vi "test9cameras.vi"() -> ()   [LabVIEW 2013]
uses:
  <vilib>/vision/Image Controls.llb/IMAQ Image.ctl
  shared programs/GUI_Template/GUI_master/tcp new data cluster.ctl
  shared programs/GUI_Template/GUI_master/tcp_new_data_event.ctl
panel:
  in  "names1":bool
  in  "MirrorsNames 2":string[](array[string])=["TS-253a_in"]
  out "image::6":T1(plugin-control) caption="Mode1"
  out "image::5":T1(plugin-control) caption="Mode1"
  out "image::4":T1(plugin-control) caption="Mode1"
  out "image::3":T1(plugin-control) caption="Mode1"
  out "image::2":T1(plugin-control) caption="Mode1"
  out "error IO 2":errorcluster
  in  "insert tag":bool=TRUE
  out "tcp data event":T2
  out "GUIdevice 1":string="M1Cam"
  out "GUIdevice 2":string="M1Cam"
  out "GUIdevice 3":string="M1Cam"
  out "GUIdevice 4":string="M1Cam"
  out "GUIdevice 5":string="M1Cam"
  out "GUIdevice 6":string="M1Cam"
  out "image::1":T1(plugin-control) caption="Mode1"
  in  "MirrorsNames":string[](array[string])=["TS-253a_in", "TS-Mode1", "StagingAlignBeam1", "StagingM1Far", "StagingM1Near", "StagingM3Far", "StagingOAP1Far", "StagingOAP1Near", "StagingOAP2Near"]
  in  "stop":bool
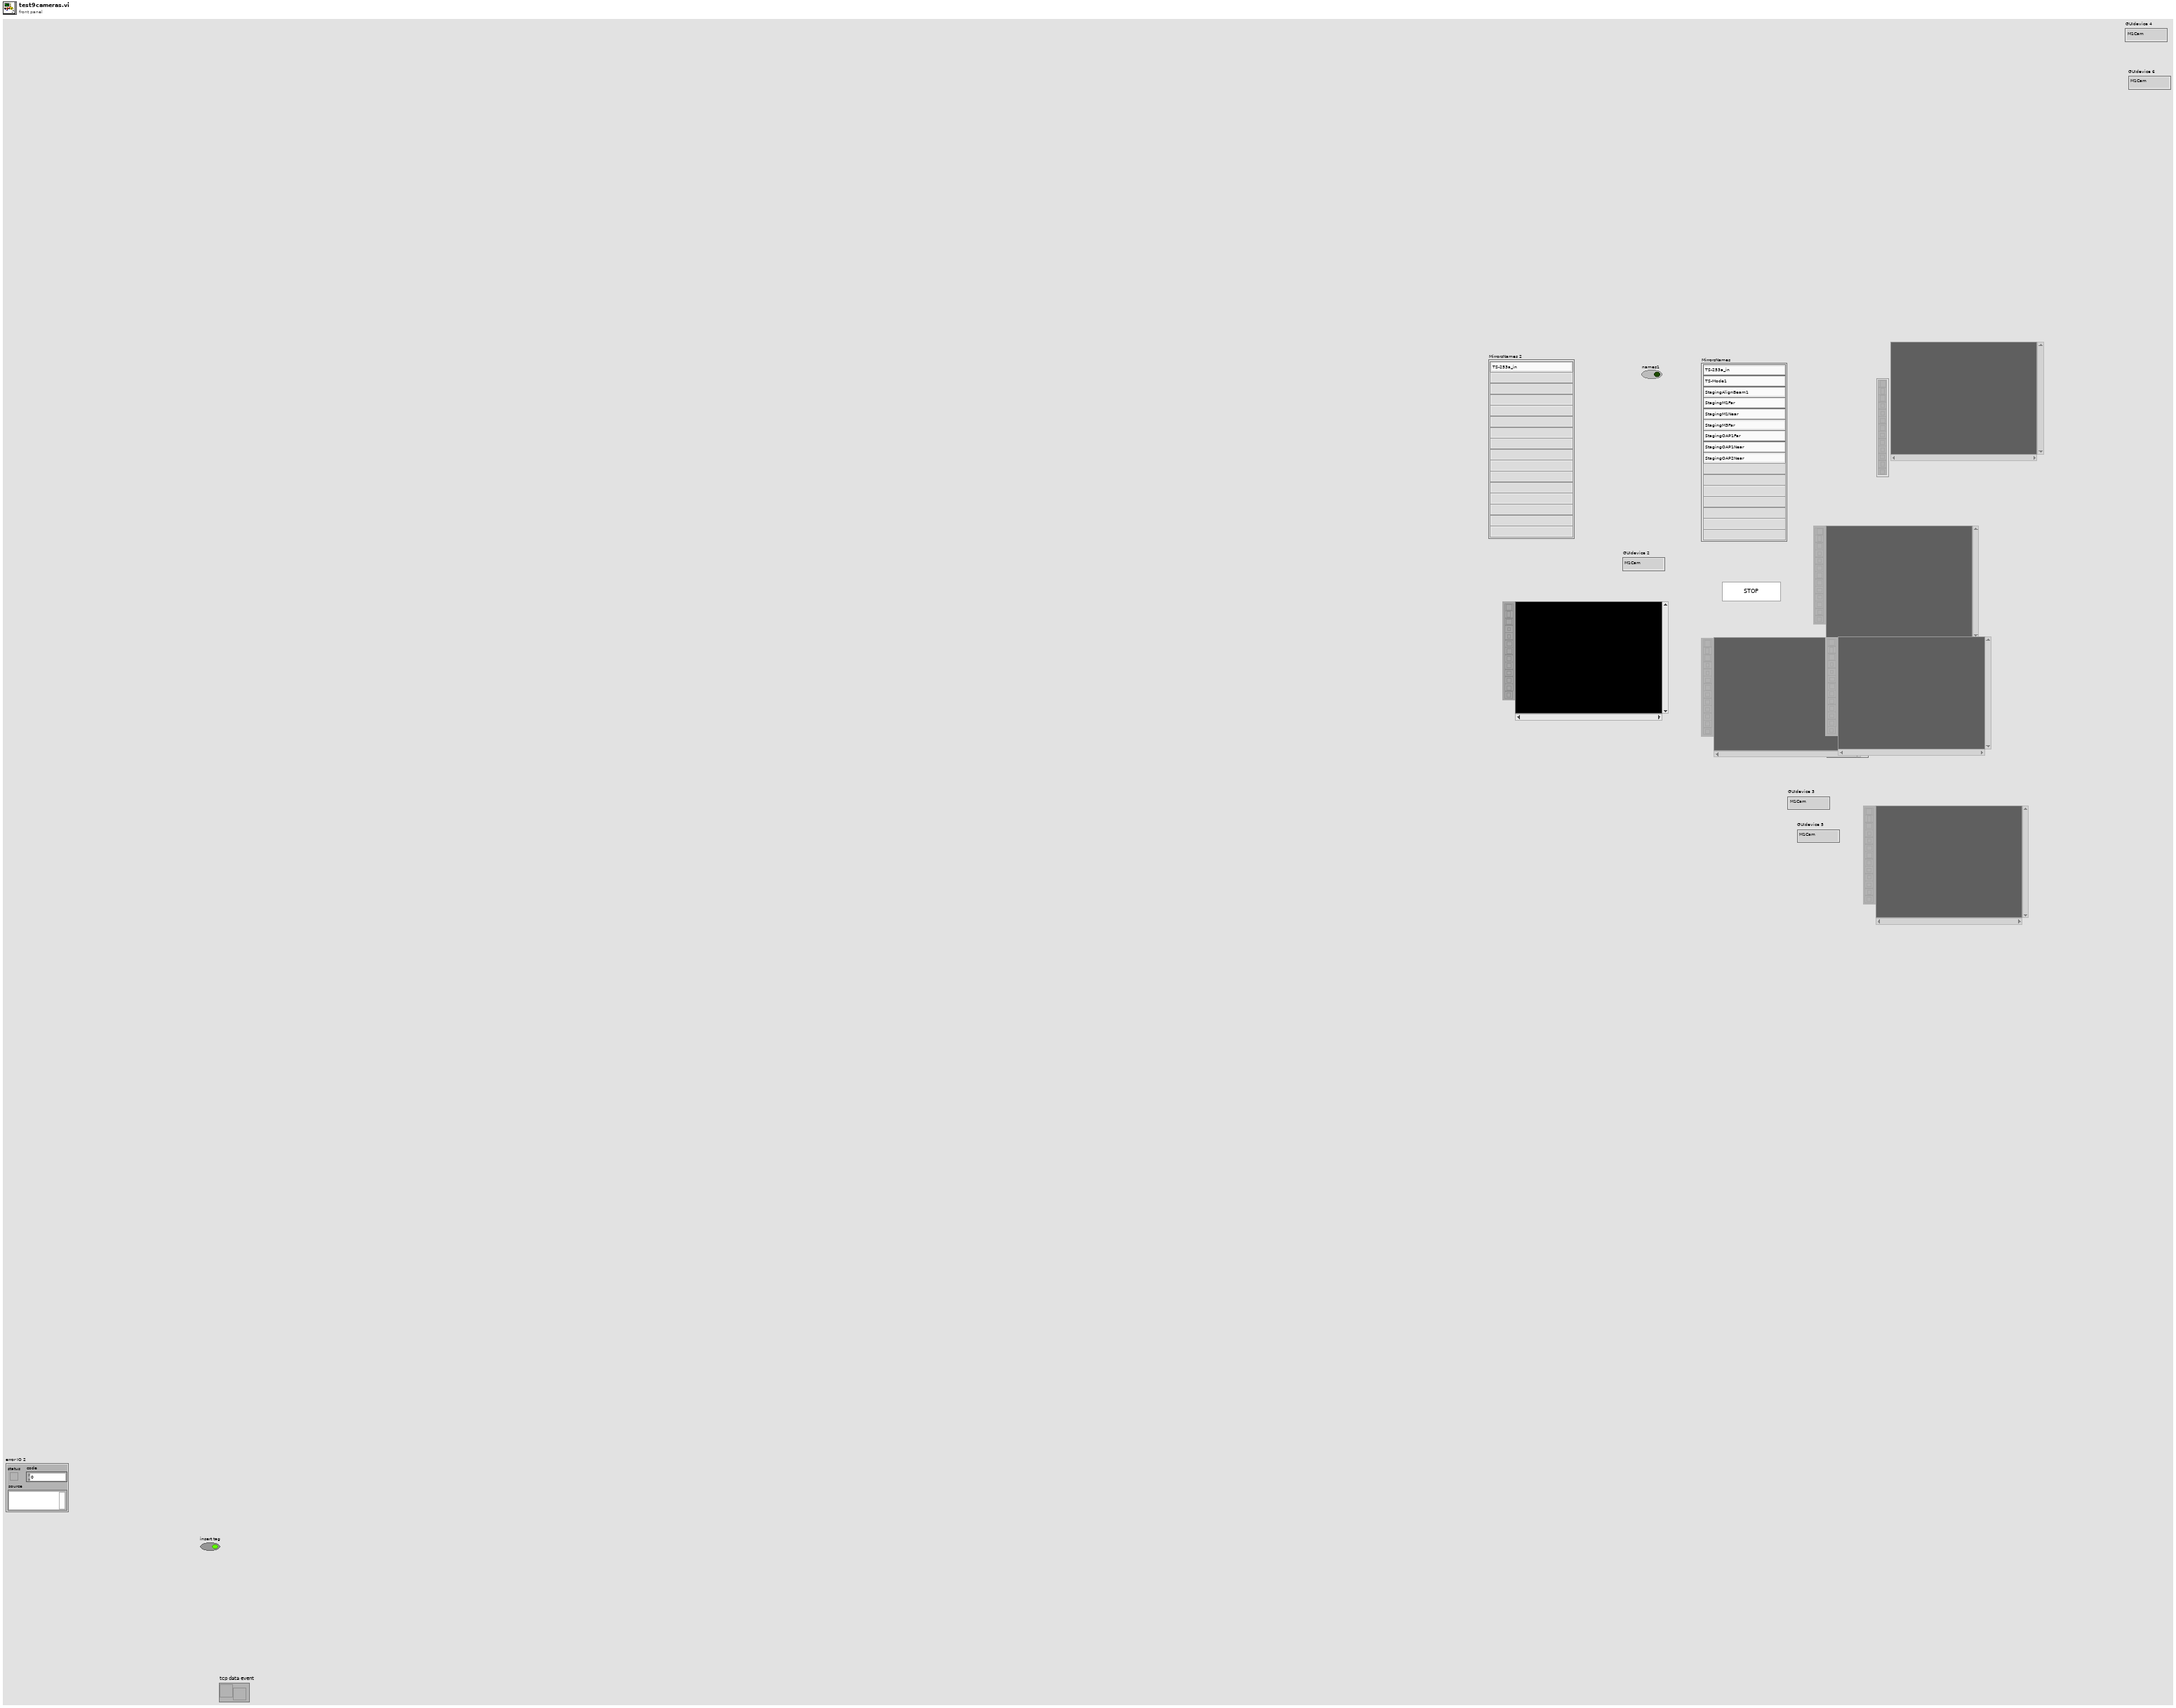
[diagram p1: front panel]
types:
  T1 = typedef "IMAQ Image.ctl" = refnum<image>
  T2 = typedef "tcp_new_data_event.ctl" = refnum<user-event>
  T3 = enum32{"invalid app kind", "Development System", "Run Time System", "Student Edition", "Embedded LabVIEW", "Evaluation", "Custom"}
  T4 = enum32{"Invalid", "Standard", "Closed", "Hidden", "Minimized", "Maximized"}
  T5 = cluster{"Core":cluster{"Current VI Reference":refnum<vi>, "Close Panel on Exit?":bool}, "Your Boolean data":bool, "Your string data":string}
  T6 = cluster{"Current VI Reference":refnum<vi>, "Close Panel on Exit?":bool}
  T7 = typedef "tcp new data cluster.ctl" = cluster{"EventEnum":enum16{"new data", "connection status update"}, "Device name":string}
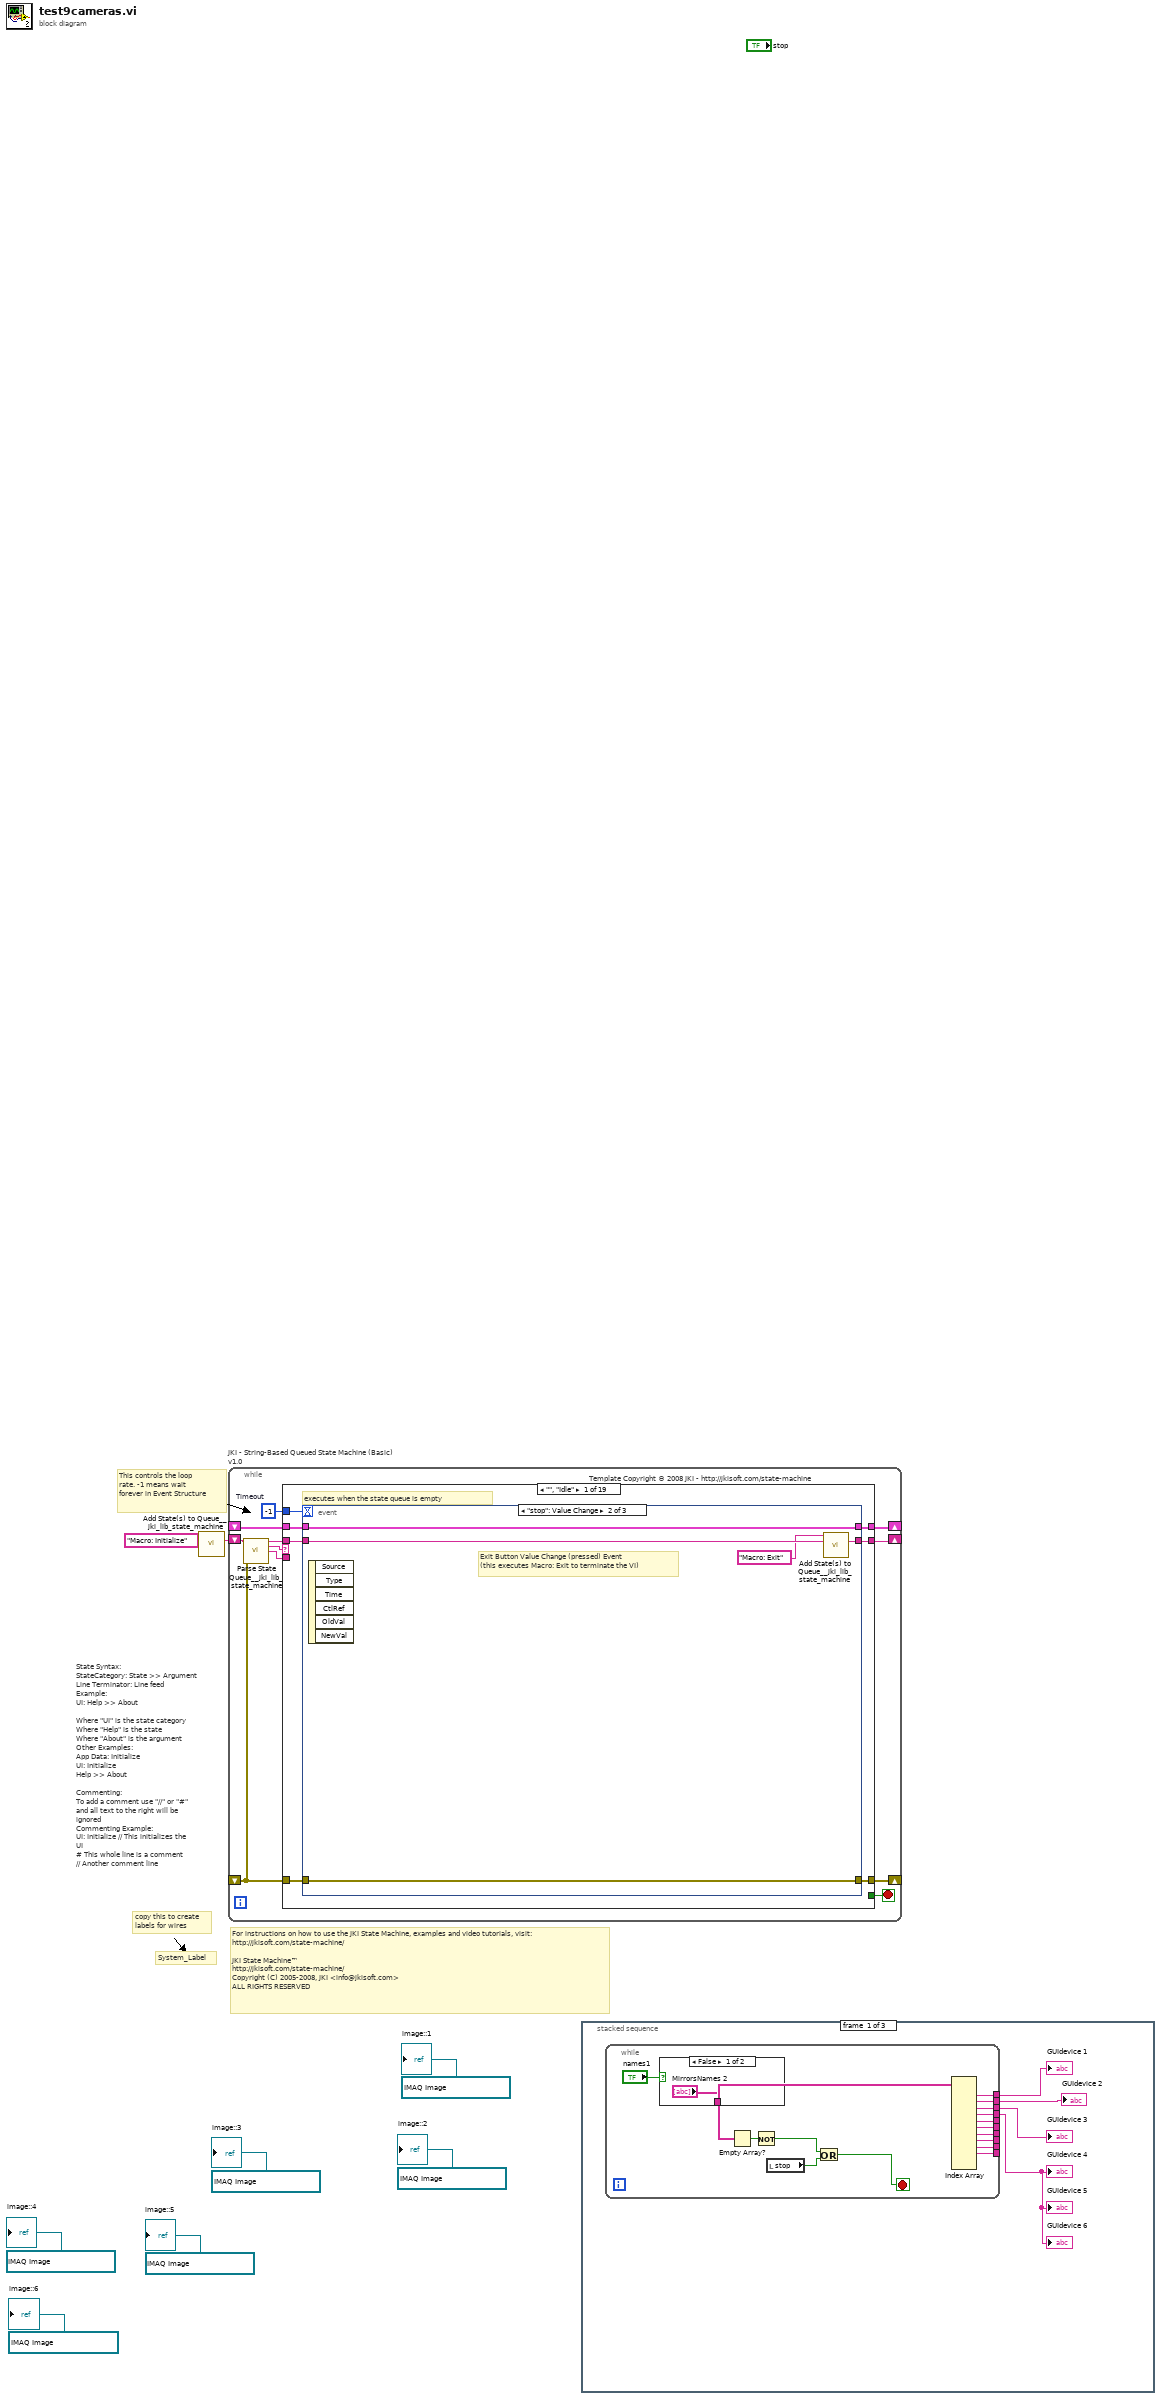
[diagram p0: block diagram]
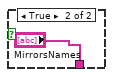
[diagram p2: hidden frame]
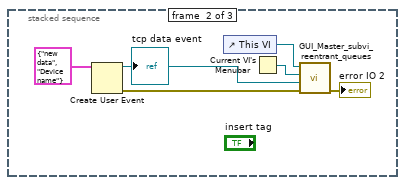
[diagram p3: hidden frame]
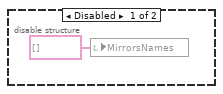
[diagram p5: hidden frame]
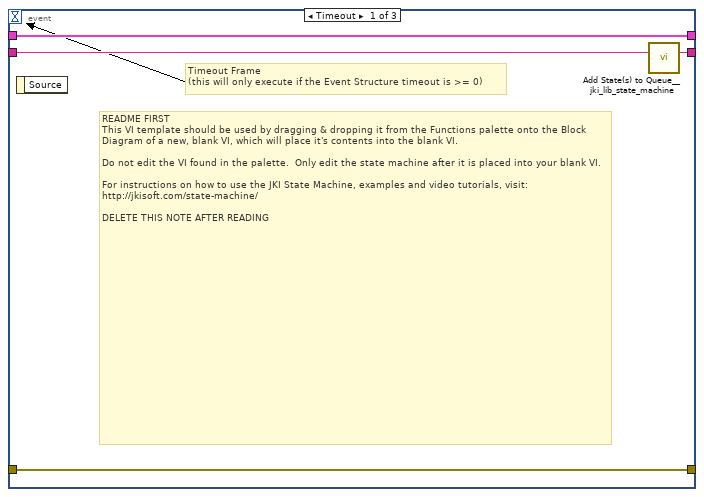
[diagram p6: hidden frame]
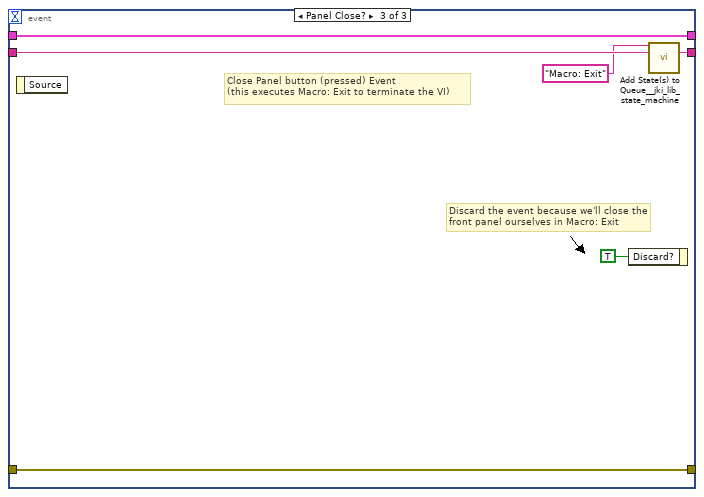
[diagram p7: hidden frame]
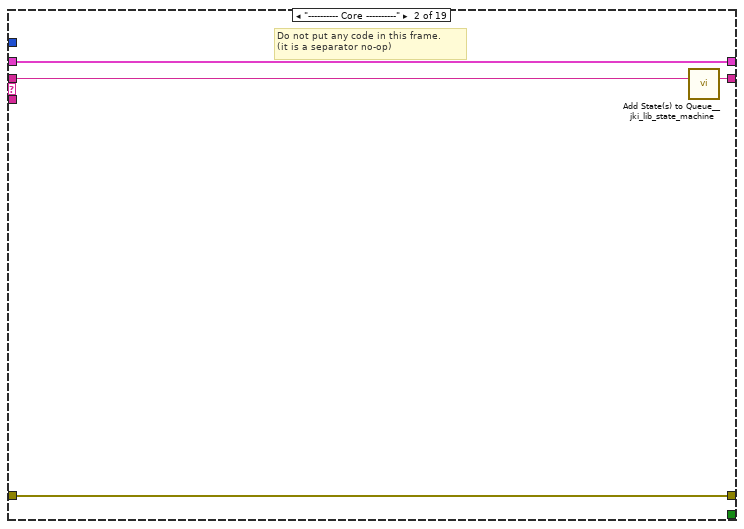
[diagram p8: hidden frame]
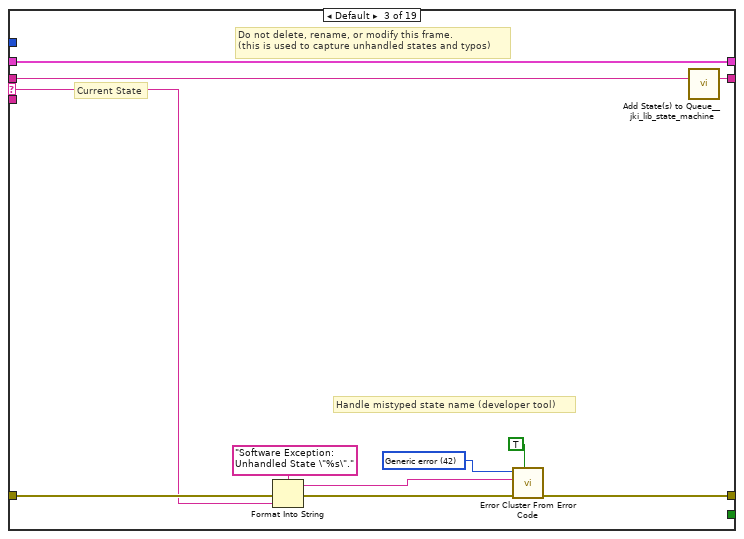
[diagram p9: hidden frame]
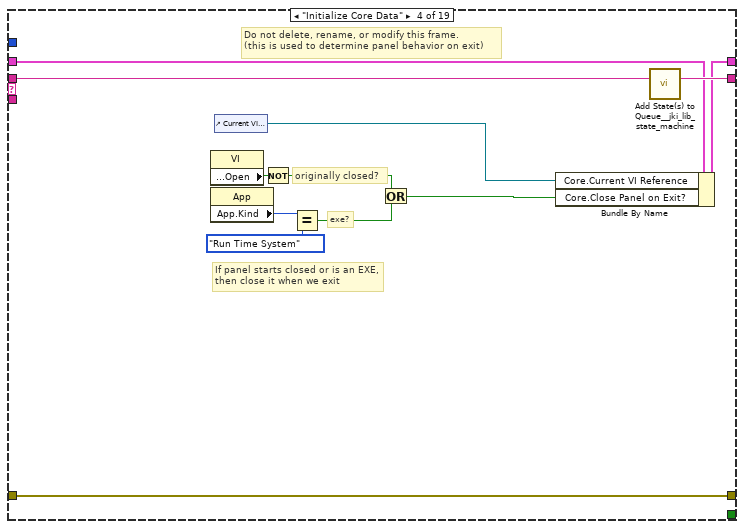
[diagram p10: hidden frame]
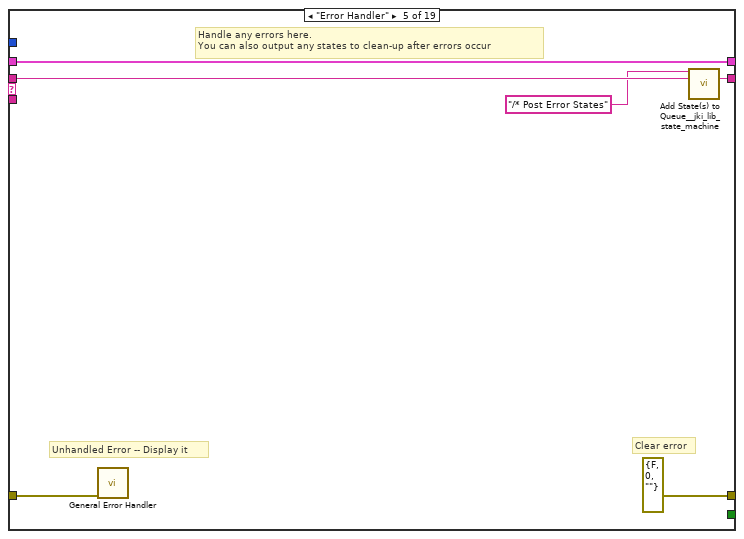
[diagram p11: hidden frame]
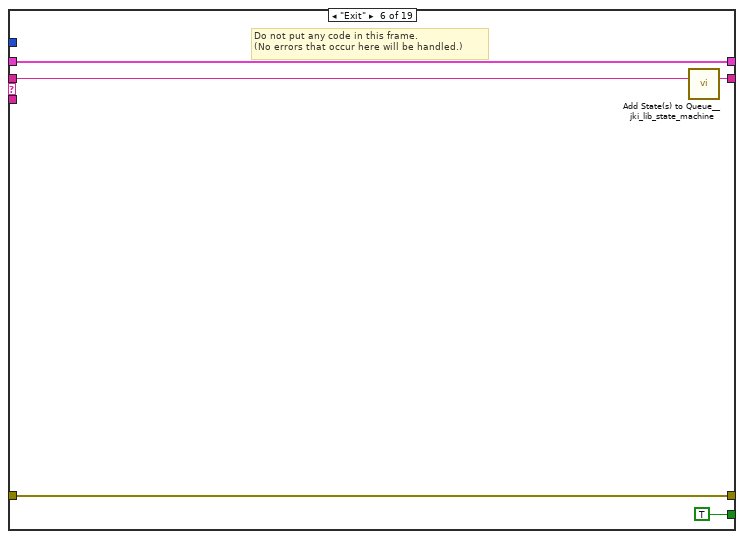
[diagram p12: hidden frame]
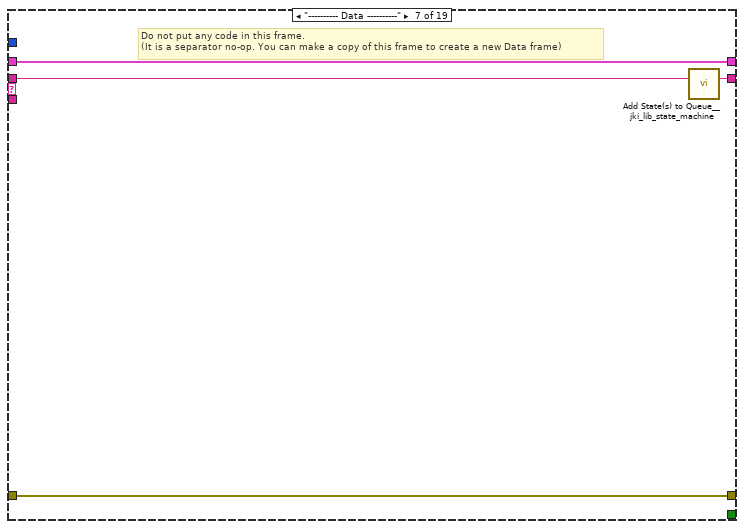
[diagram p13: hidden frame]
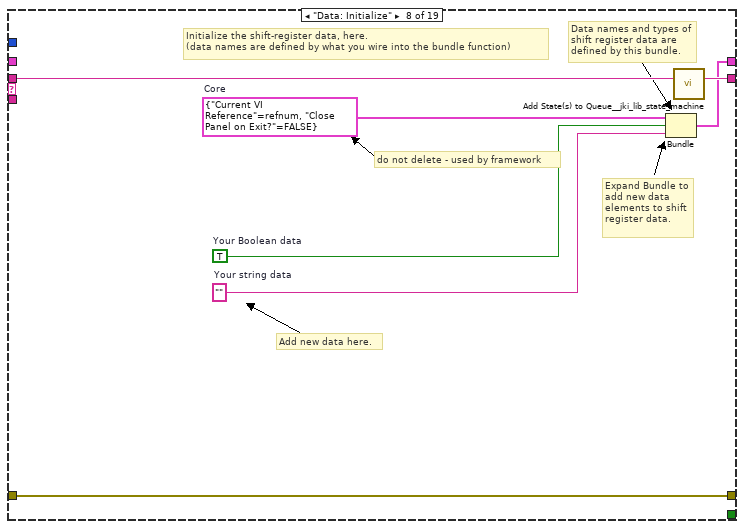
[diagram p14: hidden frame]
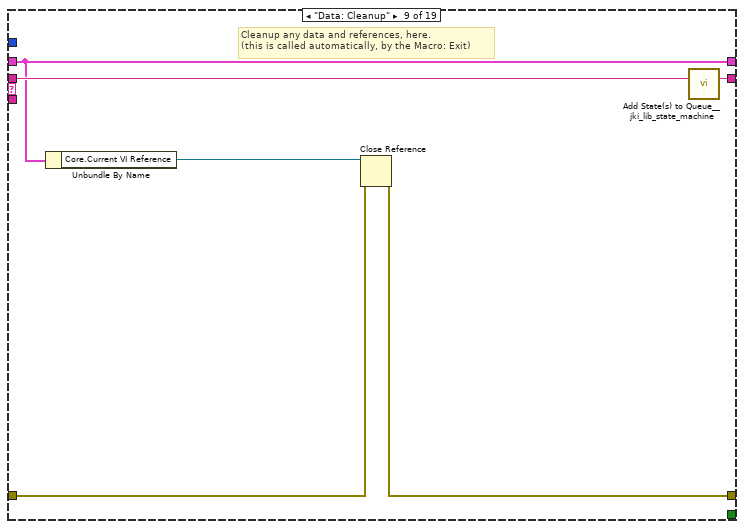
[diagram p15: hidden frame]
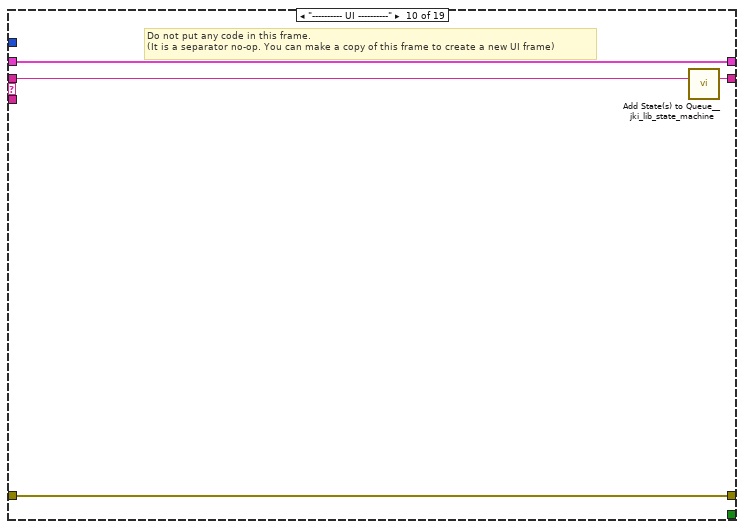
[diagram p16: hidden frame]
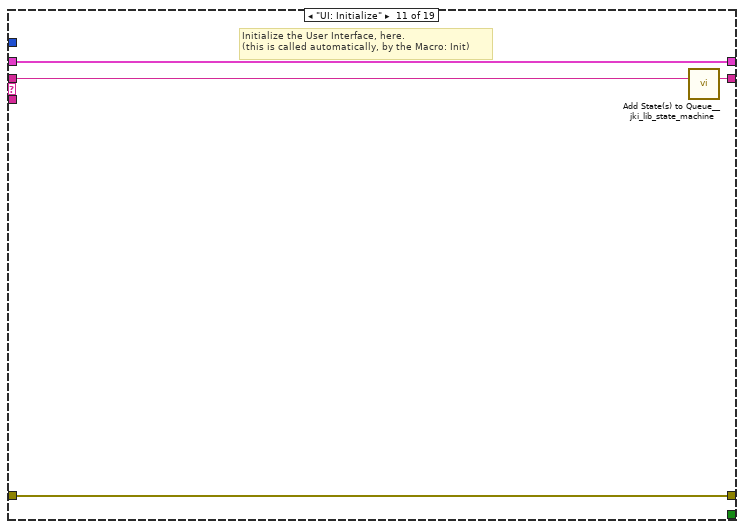
[diagram p17: hidden frame]
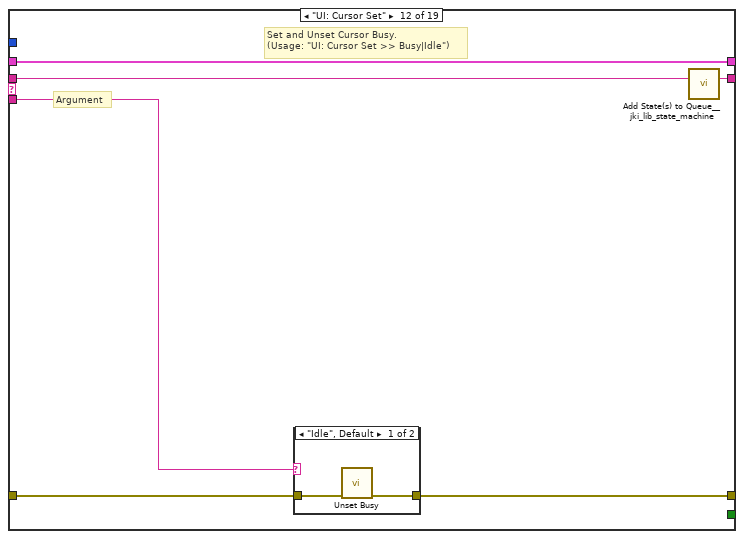
[diagram p18: hidden frame]
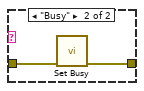
[diagram p19: hidden frame]
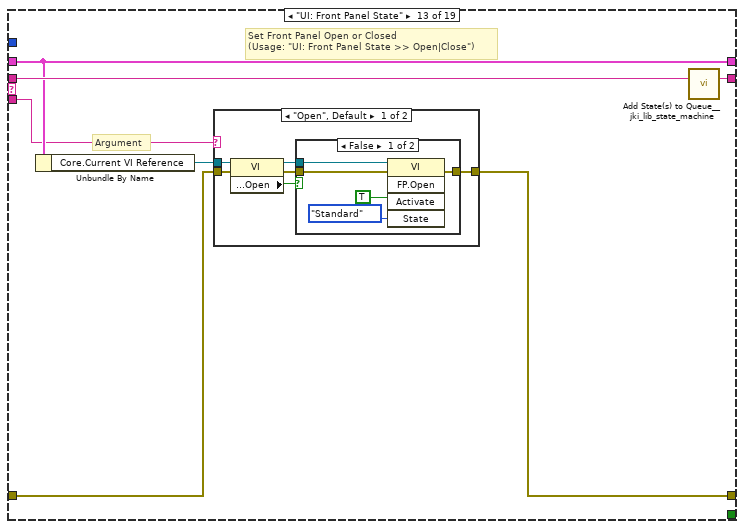
[diagram p20: hidden frame]
diagram:
  # "For instructions on how to use the JKI State Machine, examples and video tutorials, visit:\nhttp://jkisoft.com/state-machine/\n\nJKI State Machine™\nhttp://jkisoft.com/state-machine/\nCopyright (C) 2005-2008, JKI <info@jkisoft.com>\nALL RIGHTS RESERVED"
  # "State Syntax:\nStateCategory: State >> Argument\nLine Terminator: Line feed\nExample:\nUI: Help >> About\n\nWhere \"UI\" is the state category\nWhere \"Help\" is the state\nWhere \"About\" is the argument\nOther Examples:\nApp Data: Initialize\nUI: Initialize\nHelp >> About\n\nCommenting:\nTo add a comment use \"//\" or \"#\" and all text to the right will be ignored\nCommenting Example:\nUI: Initialize // This initializes the UI\n# This whole line is a comment\n// Another comment line"
  # "copy this to create labels for wires"
  # "This controls the loop rate. -1 means wait forever in Event Structure"
  # "System_Label"
  n1 = call <vilib>:"Add State(s) to Queue__jki_lib_state_machine.vi"("State(s) in (\"\")"="Macro: Initialize") -> ("States Out"=w8:string)  [unwired: 14 in]
  n2 = while "JKI - String-Based Queued State Machine (Basic) v1.0" {
    shift-right: [w12] -> _
    shift-left: _ -> [w11]
    shift-right: [w15] -> _
    shift-left: _ -> [w9]
    shift-right: [w14] -> _
    shift-left: w8 -> [w16]
    stop <- w13 stop-if-true
    w10 = -1  # Timeout
    # "Template Copyright © 2008 JKI - http://jkisoft.com/state-machine"
    n3 = call <vilib>:"Parse State Queue__jki_lib_state_machine.vi"("State Queue"=w16, "Error In (no error)"=w9) -> ("Remaining States"=w18:string, "Current State"=w19:string, "Arguments"=w17:string)  [unwired: 11 in]
    n4 = case shown="\"\", \"Idle\"" w19 {
      selector: w19 -> [_ _ w46 _ _ _ _ _ _ _ _ _ _ _ _ _ _ _ _]
      tunnel: w18 -> [w26 w45 w50 w68 w74 w79 w83 w90 w96 w100 w104 w110 w121 w147 w152 w162 w166 w170 w174]
      tunnel: w17 -> [_ _ _ _ _ _ _ _ _ _ _ w105 w115 _ _ _ _ _ _]
      tunnel: w11 -> [w24 w42 w48 w59 w71 w77 w80 _ w91 w97 w102 w108 w117 w144 w149 w159 w163 w167 w171]
      tunnel: [w23 w43 w52 w65 errorcluster {"status"=FALSE, "code"=0, "source"=""} ("error out") w76 w81 w87 w92 w98 w101 w106 w118 w145 w150 w160 w164 w168 w172] -> w15
      tunnel: w9 -> [w22 w43 w51 w65 w70 w76 w81 w87 w93 w98 w101 w107 w119 w145 w150 w160 w164 w168 w172]
      tunnel: [w25 w44 w49 w67 w73 w78 w82 w89 w95 w99 w103 w109 w120 w146 w151 w161 w165 w169 w173] -> w14
      tunnel: [_ _ _ _ _ TRUE _ _ _ _ _ _ _ _ _ _ _ _ _] -> w13
      tunnel: [w21 w42 w48 w66 w71 w77 w80 w88 w91 w97 w102 w108 w117 w144 w149 w159 w163 w167 w171] -> w12
      tunnel: w10 -> [w20 _ _ _ _ _ _ _ _ _ _ _ _ _ _ _ _ _ _]
      frame "", "Idle" {
        # "executes when the state queue is empty"
        n5 = event shown="[1] \"stop\": Value Change" {
          selector: _ -> [_ _ _]
          dyn-events: _ -> [_ _ _]
          timeout: w20 -> [_ _ _]
          tunnel: w26 -> [w30 w35 w41]
          tunnel: [w29 w34 w40] -> w25
          tunnel: w24 -> [w27 w32 w38]
          tunnel: [w28 w33 w39] -> w23
          tunnel: w22 -> [w28 w33 w39]
          tunnel: [w27 w32 w38] -> w21
          event Timeout {
            # "README FIRST\nThis VI template should be used by dragging & dropping it from the Functions palette onto the Block Diagram of a new, blank VI, which will place it's contents into the blank VI.\n\nDo not edit the VI found in the palette.  Only edit the state machine after it is placed into your blank VI.\n\nFor instructions on how to use the JKI State Machine, examples and video tutorials, visit:\nhttp://jkisoft.com/state-machine/\n\nDELETE THIS NOTE AFTER READING"
            # "Timeout Frame\n(this will only execute if the Event Structure timeout is >= 0)"
            n6 = event-data() -> ()  [unwired: 1 in, 1 out]
            n7 = call <vilib>:"Add State(s) to Queue__jki_lib_state_machine.vi"("State(s) in (\"\")"=w30) -> ("States Out"=w29:string)  [unwired: 14 in]
          }
          event "stop": Value Change {
            # "Exit Button Value Change (pressed) Event\n(this executes Macro: Exit to terminate the VI)"
            n8 = event-data() -> ()  [unwired: 1 in, 6 out]
            n9 = call <vilib>:"Add State(s) to Queue__jki_lib_state_machine.vi"("State(s) in Front (\"\")"="Macro: Exit", "State(s) in (\"\")"=w35) -> ("States Out"=w34:string)  [unwired: 13 in]
          }
          event Panel Close? {
            # "Discard the event because we'll close the front panel ourselves in Macro: Exit"
            # "Close Panel button (pressed) Event\n(this executes Macro: Exit to terminate the VI)"
            n10 = event-data() -> ()  [unwired: 1 in, 1 out]
            n11 = event-data("Discard?"=TRUE) -> ()  [unwired: 1 in, 1 out]
            n12 = call <vilib>:"Add State(s) to Queue__jki_lib_state_machine.vi"("State(s) in Front (\"\")"="Macro: Exit", "State(s) in (\"\")"=w41) -> ("States Out"=w40:string)  [unwired: 13 in]
          }
        }
      }
      frame "---------- Core ----------" {
        # "Do not put any code in this frame.\n(it is a separator no-op)"
        n13 = call <vilib>:"Add State(s) to Queue__jki_lib_state_machine.vi"("State(s) in (\"\")"=w45) -> ("States Out"=w44:string)  [unwired: 14 in]
      }
      frame Default {
        w55 = 42 items=["No error", "Argument error", "Memory is full", "Out of zone", "End of file", "File already open", "Generic file I/O error", "File not found", "File permission error", "Disk is full", "Duplicate path", "Too many files open", "System feature not enabled", "Resource file not found", "Cannot add resource", "Resource not found", "Image not found", "Image memory error", "Pen does not exist", "Config type invalid", "Config token not found", "Config parse error", "Config memory error", "Bad external code format", "Bad external code offset", "External code not present", "Null window", "Destroy window error", "Null menu", "Print aborted", "Bad print record", "Print driver error", "Windows error during printing", "Memory error during printing", "Print dialog error", "Generic print error", "Invalid device refnum", "Device not found", "Device parameter error", "Device unit error", "Cannot open device", "Device call aborted", "Generic error", "Cancelled by user", "Object ID too low", "Object ID too high", "Object not in heap", "Unknown heap", "Unknown object (invalid DefProc)", "Unknown object (DefProc not in table)", "Message out of range", "Invalid (null) method", "Unknown message", "Manager call not supported", "Bad address", "Network operation in progress", "Network operation timed out", "Connection is busy", "Network attribute not supported", "Network error", "Address in use", "System out of memory", "Connection aborted", "Connection refused", "Not connected", "Already connected", "Connection closed", "Initialization error (interapplication manager)", "Bad occurrence", "Wait on unbound occurrence handler", "Occurrence queue overflow", "Datalog type conflict", "Unused", "Unrecognized type (interapplication manager)", "Memory corrupt", "Failed to make temporary DLL", "Old CIN version", "Drag socket not found", "Failed to load drop-object", "Failed to register OLE object", "Failed to release OLE object", "Format specifier type mismatch", "Unknown format specifier", "Too few format specifiers", "Too many format specifiers", "Scan failed", "Newer CIN version", "Error converting to variant", "Runtime menu error", "Password tampered", "Variant attribute not found", "Incompatible variant data type", "Event data is not available", "Event Store is not present", "Occurrence is not found", "Event Queue is not created", "Event info is not available", "Refnum passed is NULL", "Error retrieving Class GUID", "Error retrieving CoClass GUID", "Error retrieving TypeLib GUID.", "Bad built application magic bytes.", "Specific driver is different from the specific driver associated with the Logical Name.", "There is no session opened to the class driver.", "Max Error", "MAX - Error with config objects", "MAX - Error loading configuration", "MAX - Group not supported"]
        # "Current State"
        # "Do not delete, rename, or modify this frame.\n(this is used to capture unhandled states and typos)"
        # "Handle mistyped state name (developer tool)"
        n14 = Format Into String(format string="Software Exception: Unhandled State \"%s\"." ("message"), error in=w51, w46) -> (resulting string=w54:string, error out=w53:errorcluster)  [unwired: 1 in]
        n15 = call <vilib>:"Error Cluster From Error Code.vi"("show call chain? (False)"=TRUE, "error in (no error)"=w53, "error message (\"\")"=w54, "error code (0)"=w55) -> ("error out"=w52:errorcluster)  [unwired: 5 in]
        n16 = call <vilib>:"Add State(s) to Queue__jki_lib_state_machine.vi"("State(s) in (\"\")"=w50) -> ("States Out"=w49:string)  [unwired: 14 in]
      }
      frame "Initialize Core Data" {
        # "Do not delete, rename, or modify this frame.\n(this is used to determine panel behavior on exit)"
        # "originally closed?"
        # "exe?"
        # "If panel starts closed or is an EXE, then close it when we exit"
        n17 = property class="VI"() -> ("Front Panel.Open"=w64:bool)  [unwired: 2 in, 2 out]
        n18 = property class="App"() -> ("App.Kind"=w63:T3)  [unwired: 2 in, 2 out]
        n19 = control-ref of="Current VI Reference"() -> (w57:refnum<vi>)
        n20 = Not(x=w64) -> (.not. x?=w61:bool)
        n21 = Equal?(x=w63, y=T3."Run Time System" ("Application:Kind")) -> (x = y?=w60:bool)
        n22 = Or(x=w61, y=w60) -> (x .or. y?=w58:bool)
        n23 = Bundle By Name(cluster=w59, "Core.Current VI Reference"=w57, "Core.Close Panel on Exit?"=w58) -> (w66:T5)
        n24 = call <vilib>:"Add State(s) to Queue__jki_lib_state_machine.vi"("State(s) in (\"\")"=w68) -> ("States Out"=w67:string)  [unwired: 14 in]
      }
      frame "Error Handler" {
        # "Unhandled Error -- Display it"
        # "Handle any errors here.\nYou can also output any states to clean-up after errors occur"
        # "Clear error"
        n25 = call <vilib>:"General Error Handler.vi"("error in (no error)"=w70) -> ()  [unwired: 10 in, 5 out]
        n26 = call <vilib>:"Add State(s) to Queue__jki_lib_state_machine.vi"("State(s) in Front (\"\")"="/* Post Error States", "State(s) in (\"\")"=w74) -> ("States Out"=w73:string)  [unwired: 13 in]
      }
      frame "Exit" {
        # "Do not put any code in this frame.\n(No errors that occur here will be handled.)"
        n27 = call <vilib>:"Add State(s) to Queue__jki_lib_state_machine.vi"("State(s) in (\"\")"=w79) -> ("States Out"=w78:string)  [unwired: 14 in]
      }
      frame "---------- Data ----------" {
        # "Do not put any code in this frame.\n(It is a separator no-op. You can make a copy of this frame to create a new Data frame)"
        n28 = call <vilib>:"Add State(s) to Queue__jki_lib_state_machine.vi"("State(s) in (\"\")"=w83) -> ("States Out"=w82:string)  [unwired: 14 in]
      }
      frame "Data: Initialize" {
        w84 = T6 {"Current VI Reference"=refnum, "Close Panel on Exit?"=FALSE}  # Core
        w86 = TRUE  # Your Boolean data
        w85 = ""  # Your string data
        # "do not delete - used by framework"
        # "Expand Bundle to add new data elements to shift register data."
        # "Add new data here."
        # "Data names and types of shift register data are defined by this bundle."
        # "Initialize the shift-register data, here.\n(data names are defined by what you wire into the bundle function)"
        n29 = Bundle("Core"=w84, "Your Boolean data"=w86, "Your string data"=w85) -> (w88:T5)  [unwired: 1 in]
        n30 = call <vilib>:"Add State(s) to Queue__jki_lib_state_machine.vi"("State(s) in (\"\")"=w90) -> ("States Out"=w89:string)  [unwired: 14 in]
      }
      frame "Data: Cleanup" {
        # "Cleanup any data and references, here.\n(this is called automatically, by the Macro: Exit)"
        n31 = Unbundle By Name(w91) -> ("Core.Current VI Reference"=w94:refnum<vi>)
        n32 = Close Reference(reference=w94, error in (no error)=w93) -> (error out=w92:errorcluster)
        n33 = call <vilib>:"Add State(s) to Queue__jki_lib_state_machine.vi"("State(s) in (\"\")"=w96) -> ("States Out"=w95:string)  [unwired: 14 in]
      }
      frame "---------- UI ----------" {
        # "Do not put any code in this frame.\n(It is a separator no-op. You can make a copy of this frame to create a new UI frame)"
        n34 = call <vilib>:"Add State(s) to Queue__jki_lib_state_machine.vi"("State(s) in (\"\")"=w100) -> ("States Out"=w99:string)  [unwired: 14 in]
      }
      frame "UI: Initialize" {
        # "Initialize the User Interface, here.\n(this is called automatically, by the Macro: Init)"
        n35 = call <vilib>:"Add State(s) to Queue__jki_lib_state_machine.vi"("State(s) in (\"\")"=w104) -> ("States Out"=w103:string)  [unwired: 14 in]
      }
      frame "UI: Cursor Set" {
        # "Argument"
        # "Set and Unset Cursor Busy.\n(Usage: \"UI: Cursor Set >> Busy|Idle\")"
        n36 = case shown="\"Idle\", Default" w105 {
          tunnel: w107 -> [w112 w114]
          tunnel: [w111 w113] -> w106
          frame "Idle", Default {
            n37 = call <vilib>:"Unset Busy.vi"("error in (no error)"=w112) -> ("error out"=w111:errorcluster)  [unwired: 10 in]
          }
          frame "Busy" {
            n38 = call <vilib>:"Set Busy.vi"("error in (no error)"=w114) -> ("error out"=w113:errorcluster)  [unwired: 9 in, 1 out]
          }
        }
        n39 = call <vilib>:"Add State(s) to Queue__jki_lib_state_machine.vi"("State(s) in (\"\")"=w110) -> ("States Out"=w109:string)  [unwired: 14 in]
      }
      frame "UI: Front Panel State" {
        # "Argument"
        # "Set Front Panel Open or Closed\n(Usage: \"UI: Front Panel State >> Open|Close\")"
        n40 = Unbundle By Name(w117) -> ("Core.Current VI Reference"=w116:refnum<vi>)
        n41 = case shown="\"Open\", Default" w115 {
          tunnel: w119 -> [w125 w138]
          tunnel: [w127 w139] -> w118
          tunnel: w116 -> [w126 w136]
          frame "Open", Default {
            n42 = property class="VI"(reference=w126, error in=w125) -> (reference out=w123:refnum<vi>, error out=w124:errorcluster, "Front Panel.Open"=w122:bool)
            n43 = case shown="False" w122 {
              tunnel: [w130 w133] -> w127
              tunnel: w124 -> [w129 w133]
              tunnel: w123 -> [w128 _]
              frame False {
                n44 = invoke class="VI" method="FP.Open"(reference=w128, error in=w129, "Activate"=TRUE, "State"=T4."Standard") -> (error out=w130:errorcluster)  [unwired: 1 in, 4 out]
              }
              frame True {
              }
            }
          }
          frame "Close" {
            n45 = property class="VI"(reference=w136, error in=w138) -> (reference out=w135:refnum<vi>, error out=w137:errorcluster, "Front Panel.Open"=w134:bool)
            n46 = case shown="True" w134 {
              tunnel: [w140 w143] -> w139
              tunnel: w137 -> [w140 w142]
              tunnel: w135 -> [_ w141]
              frame False {
              }
              frame True {
                n47 = invoke class="VI" method="FP.Close"(reference=w141, error in=w142) -> (error out=w143:errorcluster)  [unwired: 1 in, 2 out]
              }
            }
          }
        }
        n48 = call <vilib>:"Add State(s) to Queue__jki_lib_state_machine.vi"("State(s) in (\"\")"=w121) -> ("States Out"=w120:string)  [unwired: 14 in]
      }
      frame "---------- Macro ----------" {
        # "Do not put any code in this frame.\n(It is a separator no-op. You can make a copy of this frame to create a new Macro frame)"
        n49 = call <vilib>:"Add State(s) to Queue__jki_lib_state_machine.vi"("State(s) in (\"\")"=w147) -> ("States Out"=w146:string)  [unwired: 14 in]
      }
      frame "Macro: Initialize" {
        w148 = "Data: Initialize\nInitialize Core Data\nUI: Initialize\nUI: Front Panel State >> Open"  # Data: Initialize Initialize Core Data UI: Initialize UI: Front Panel State >> Open
        # "Initialization Macro\n(This is called once, when the VI starts)"
        n50 = call <vilib>:"Add State(s) to Queue__jki_lib_state_machine.vi"("State(s) in Front (\"\")"=w148, "State(s) in (\"\")"=w152) -> ("States Out"=w151:string)  [unwired: 13 in]
      }
      frame "Macro: Exit" {
        # "Exit Macro\n(This is called once, when the VI exits)"
        n51 = Unbundle By Name(w159) -> ("Core.Close Panel on Exit?"=w158:bool)
        n52 = Select(t="UI: Front Panel State >> Close", s=w158, f="") -> (s? t:f=w155:string)
        n53 = call <vilib>:"Add State(s) to Queue__jki_lib_state_machine.vi"("State(s) in (\"\")"=w155, "State(s) at Back (\"\")"="Data: Cleanup\nExit") -> ("States Out"=w153:string)  [unwired: 13 in]
        n54 = call <vilib>:"Add State(s) to Queue__jki_lib_state_machine.vi"("State(s) in Front (\"\")"=w153, "State(s) in (\"\")"=w162) -> ("States Out"=w161:string)  [unwired: 13 in]
      }
      frame "---------- New Category ----------" {
        # "Template Separator\n(You can make a copy of, or modify, this frame)"
        n55 = call <vilib>:"Add State(s) to Queue__jki_lib_state_machine.vi"("State(s) in (\"\")"=w166) -> ("States Out"=w165:string)  [unwired: 14 in]
      }
      frame "New Category: 1" {
        # "Your code here.\n(You can make a copy of, or modify, this frame)"
        n56 = call <vilib>:"Add State(s) to Queue__jki_lib_state_machine.vi"("State(s) in (\"\")"=w170) -> ("States Out"=w169:string)  [unwired: 14 in]
      }
      frame "New Category: 2" {
        # "Your code here.\n(You can make a copy of, or modify, this frame)"
        n57 = call <vilib>:"Add State(s) to Queue__jki_lib_state_machine.vi"("State(s) in (\"\")"=w174) -> ("States Out"=w173:string)  [unwired: 14 in]
      }
    }
  }
  n58 = stacked-sequence {
    frame #0 {
      n59 = while {
        tunnel: [w191] -> w178
        tunnel: [w189] -> w177
        tunnel: [w188] -> w176
        tunnel: [w187] -> w175
        tunnel: [w186] -> _
        tunnel: [w185] -> _
        tunnel: [w184] -> _
        tunnel: [w183] -> _
        tunnel: [w182] -> _
        tunnel: [w181] -> _
        stop <- w192 stop-if-true
        n60 = case shown="False" "names1" {
          tunnel: ["MirrorsNames 2" "MirrorsNames"] -> w180
          frame False {
          }
          frame True {
          }
        }
        n61 = Empty Array?(array=w180) -> (empty?=w194:bool)
        n62 = Not(x=w194) -> (.not. x?=w193:bool)
        n63 = local read "stop"() -> (w190:bool)
        n64 = Or(x=w193, y=w190) -> (x .or. y?=w192:bool)
        n65 = Index Array(array=w180) -> (element #1=w191:string, element #2=w189:string, element #3=w188:string, element #4=w187:string, element #5=w186:string, element #6=w185:string, element #7=w184:string, element #8=w183:string, element #9=w182:string, element #10=w181:string)  [unwired: 12 in, 2 out]
      }
      "GUIdevice 1" <- w178
      "GUIdevice 2" <- w177
      "GUIdevice 3" <- w176
      "GUIdevice 4" <- w175
      "GUIdevice 5" <- w175
      "GUIdevice 6" <- w175
    }
    frame #1 {
      n66 = Create User Event(user event datatype=T7 {"EventEnum"=enum."new data", "Device name"="Device name"} ("New Event")) -> (user event=w197:refnum<user-event>, error out=w198:errorcluster)  [unwired: 1 in]
      "tcp data event" <- w197
      n67 = control-ref of="This VI"() -> (w201:refnum<vi>)
      n68 = Current VI's Menubar() -> (w200:refnum<k9>)
      n69 = call "GUI_Master_subvi_reentrant_queues.vi"("error in (no error)"=w198, "tcp data event"=w197, "Caller menu reference"=w200, "Caller VI ref"=w201) -> ("error out"=→"error IO 2":errorcluster)  [unwired: 7 in]
    }
    frame #2 {
      n70 = disable-structure shown="Enabled" {
        frame Disabled {
          n71 = local write "MirrorsNames"(string[] [] ("MirrorsNames")) -> ()
        }
        frame Enabled {
        }
      }
    }
  }
  "image::1" <- T1 refnum ("New Image")
  "image::2" <- T1 refnum ("New Image")
  "image::3" <- T1 refnum ("New Image")
  "image::4" <- T1 refnum ("New Image")
  "image::5" <- T1 refnum ("New Image")
  "image::6" <- T1 refnum ("New Image")
